vi "Init Scoring.vi"(8 "error in (no error)":errorcluster, 11 "SOL-Server in":refnum<class "SOL-Server.lvclass">) -> (0 "error out":errorcluster, 3 "SOL-Server out":refnum<class "SOL-Server.lvclass">)   [LabVIEW 2020, in "Summer of LabVIEW.lvlib" / "SOL-Server.lvclass"]
uses:
  SOL-Server.lvclass
  SOL-Server.lvclass/SOL-Server.ctl
  Scorer/Scorer.lvclass
  Submission/Submission.lvclass
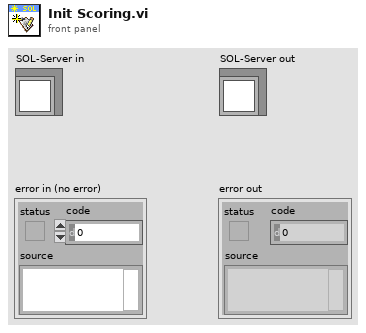
[diagram p1: front panel]
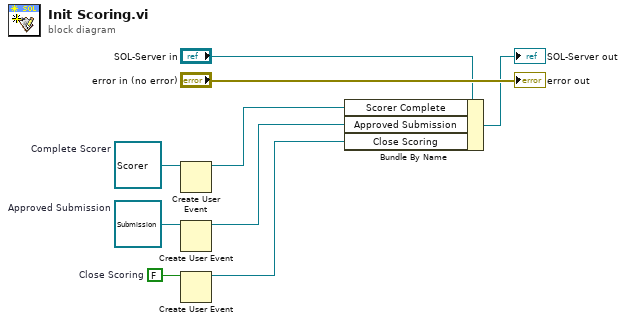
[diagram p0: block diagram]
diagram:
  w2 = FALSE  # Close Scoring
  w4 = refnum<class "Submission.lvclass"> refnum  # Approved Submission
  w8 = refnum<class "Scorer.lvclass"> refnum  # Complete Scorer
  n1 = Create User Event(user event datatype=w8) -> (user event=w7:refnum<user-event>)  [unwired: 1 in, 1 out]
  n2 = Create User Event(user event datatype=w4) -> (user event=w3:refnum<user-event>)  [unwired: 1 in, 1 out]
  n3 = Create User Event(user event datatype=w2) -> (user event=w1:refnum<user-event>)  [unwired: 1 in, 1 out]
  n4 = Bundle By Name(cluster="SOL-Server in", "Scorer Complete"=w7, "Approved Submission"=w3, "Close Scoring"=w1) -> (→"SOL-Server out":refnum<class "SOL-Server.lvclass">)
  "error out" <- "error in (no error)"
